vi "Set Unit ID Property.vi"(8 "error in (no error)":errorcluster, 10 "unit ID":u8, 11 "Modbus master in":refnum<class "Modbus Master.lvclass">) -> (0 "error out":errorcluster, 3 "Modbus master out":refnum<class "Modbus Master.lvclass">)   [LabVIEW 2020, in "Modbus Master.lvclass"]
doc: "<B>Unit ID</B> specifies the identification of a serial Modbus slave. You can use a Modbus master instance to perform read and write operations on this Modbus slave. The Property Node ignores requests from TCP Modbus master instances."
uses:
  <vilib>/Modbus/master/Modbus Master.lvclass
  C:/builds/penguin/iak/lvdsc/trunk/20.0/lv/vi.lib/Modbus/subvis/Modbus API/Modbus API.lvclass
  <vilib>/Modbus/subvis/Modbus API/Modbus API.lvclass/Modbus API.ctl
  <vilib>/Modbus/subvis/Transmission Data Unit (ADU)/Transmission Data Unit/Transmission Data Unit.lvclass/Transmission Data Unit.ctl
  <vilib>/Modbus/subvis/Transmission Data Unit (ADU)/Transmission Data Unit/Transmission Data Unit.lvclass
  <vilib>/Modbus/subvis/Modbus API/Modbus API.lvclass
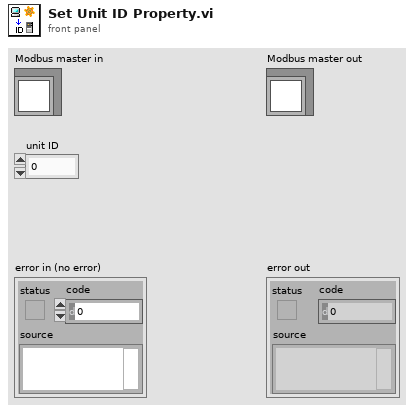
[diagram p1: front panel]
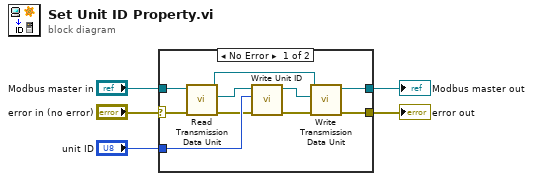
[diagram p0: block diagram]
diagram:
  n1 = case shown="No Error" "error in (no error)" {
    selector: "error in (no error)" -> [w6 w16]
    tunnel: "unit ID" -> [w15 _]
    tunnel: "Modbus master in" -> [w14 w17]
    tunnel: [w12 w17] -> w3
    tunnel: [w7 w16] -> w2
    frame No Error {
      n2 = call <vilib>:"Read Transmission Data Unit.vi"("error in (no error)"=w6, "Modbus instance in"=w14) -> ("error out"=w8:errorcluster, "transmission data unit"=w11:refnum<class "Transmission Data Unit.lvclass">, "Modbus instance out"=w13:refnum<class "Modbus Master.lvclass">)  [unwired: 7 in]
      n3 = call <vilib>:"Write Unit ID.vi"("error in (no error)"=w8, "unit ID"=w15, "transmission data unit in"=w11) -> ("error out"=w9:errorcluster, "transmission data unit out"=w10:refnum<class "Transmission Data Unit.lvclass">)  [unwired: 7 in]
      n4 = call <vilib>:"Write Transmission Data Unit.vi"("error in (no error)"=w9, "transmission data unit"=w10, "Modbus instance in"=w13) -> ("error out"=w7:errorcluster, "Modbus instance out"=w12:refnum<class "Modbus Master.lvclass">)  [unwired: 7 in]
    }
    frame Error {
    }
  }
  "error out" <- w2
  "Modbus master out" <- w3
